vi "Send Update Energy Storage Measurement.vi"(7 "Message Priority (Normal)":T3=enum."Normal", 8 "error in":errorcluster, 10 "Energy Storage Measurement":T1, 11 "Message Enqueuer":refnum<class "Message Enqueuer.lvclass">) -> (0 "error out":errorcluster, 3 "Message Enqueuer out":refnum<class "Message Enqueuer.lvclass">)   [LabVIEW 2016, in "Optimization Framework.lvlib" / "Update Energy Storage Measurement Msg.lvclass"]
doc: "This VI sends the message to an actor."
uses:
  Update Energy Storage Measurement Msg.lvclass
  <vilib>/ActorFramework/Message Enqueuer/Message Enqueuer.lvclass
  <vilib>/ActorFramework/Message Enqueuer/Message Priority.ctl
  Optimization/Controls/Measurement Cluster Energy Storage.ctl
  Optimization/Controls/3-phase Cluster.ctl
  C:/Program Files (x86)/National Instruments/LabVIEW 2016/vi.lib/ActorFramework/Message/Message.lvclass
  Update Energy Storage Measurement Msg.lvclass/Update Energy Storage Measurement Msg.ctl
  <vilib>/ActorFramework/Message Enqueuer/Message Enqueuer.lvclass/Message Enqueuer.ctl
  <vilib>/ActorFramework/Message Priority Queue/Priority Enqueue.vi
  Optimization/Optimization.lvclass
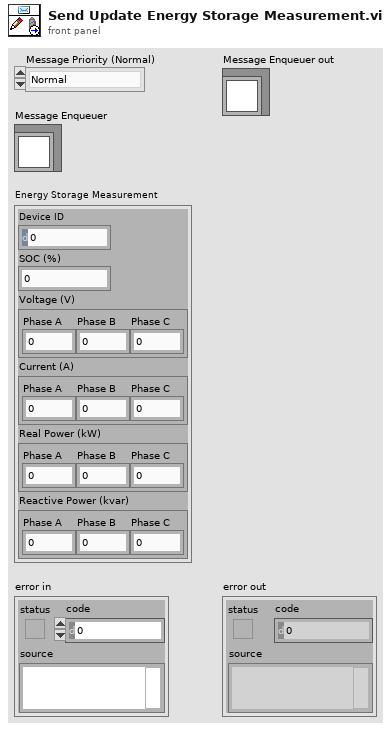
[diagram p1: front panel]
types:
  T1 = typedef "Optimization Framework.lvlib/Optimization.lvclass/Measurement Cluster Energy Storage.ctl" = cluster{"Device ID":u64, "SOC":dbl, "Voltage":T2, "Current":T2, "Real Power":T2, "Reactive Power":T2}
  T2 = typedef "Optimization Framework.lvlib/Optimization.lvclass/3-phase Cluster.ctl" = cluster{"Phase A":dbl, "Phase B":dbl, "Phase C":dbl}
  T3 = typedef "Actor Framework.lvlib/Message Enqueuer.lvclass/Message Priority.ctl" = enum16{"Low", "Normal", "High"}
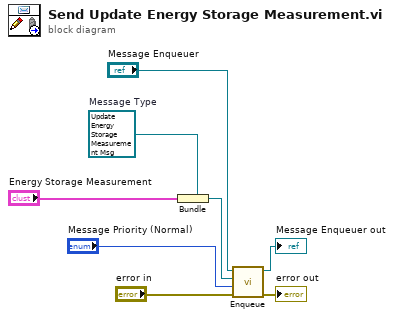
[diagram p0: block diagram]
diagram:
  w5 = refnum<class "Update Energy Storage Measurement Msg.lvclass"> refnum  # Message Type
  n1 = Bundle(cluster=w5, "Energy Storage Measurement") -> (w4:refnum<class "Update Energy Storage Measurement Msg.lvclass">)
  n2 = call <vilib>:"Enqueue.vi"("error in (no error)"="error in", "Message Priority (Normal)"="Message Priority (Normal)", "Message"=w4, "Message Enqueuer in"="Message Enqueuer") -> ("error out"=→"error out":errorcluster, "Message Enqueuer out"=→"Message Enqueuer out":refnum<class "Message Enqueuer.lvclass">)  [unwired: 6 in]
